vi "全局变量测试.vi"() -> ()   [LabVIEW 2020]
panel:
  out "地址： 2":string
  out "电话： 2":string
  in  "地址：":string
  in  "电话：":string
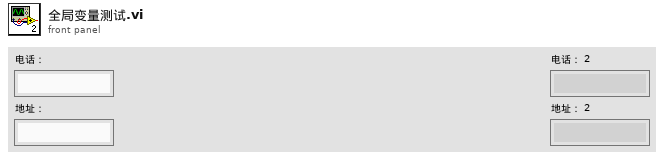
[diagram p1: front panel]
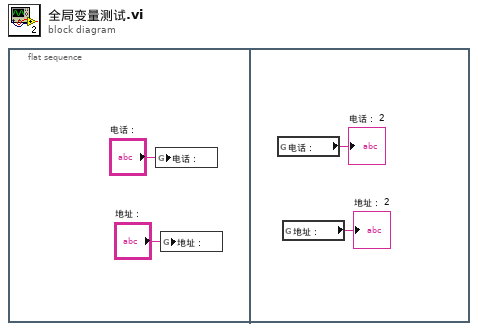
[diagram p0: block diagram]
diagram:
  n1 = flat-sequence {
    frame #0 {
      n2 = global write "快捷购买信息.vi" "电话："("电话：") -> ()
      n3 = global write "快捷购买信息.vi" "地址："("地址：") -> ()
    }
    frame #1 {
      n4 = global read "快捷购买信息.vi" "电话："() -> (→"电话： 2":string)
      n5 = global read "快捷购买信息.vi" "地址："() -> (→"地址： 2":string)
    }
  }
